vi "Get Stream State Register.vi"(6 "ready for output":bool=TRUE, 7 "stream state register":T2) -> (1 "output updated":bool caption="output valid", 2 "stream.state":T1)   [LabVIEW 2015, in "niInstr Streaming v1 FPGA.lvlib"]
uses:
  <instrlib>/_niInstr/Streaming/v1/FPGA/niInstr Streaming v1 FPGA.lvlib
  <instrlib>/_niInstr/Streaming/v1/FPGA/Public/Stream State Register.ctl
  <instrlib>/_niInstr/Streaming/v1/Common/Stream State.ctl
  <vilib>/rvi/Emulation/niFpgaSctlEmulationGetInTimedLoop.vi
  <vilib>/rvi/DataTransferAndStorage/Container/Common/niFpgaContainerExecOnDevCompGetState.vi
  <vilib>/rvi/Emulation/niFpgaEmulationIsFPGAContextNoSignature.vi
  <vilib>/rvi/DataTransferAndStorage/Container/Common/niFpgaContainerGetUniqueNameForEmu.vi
  <vilib>/rvi/eio/common/nirviEmuReportErrorAndStop.vi
  <vilib>/rvi/Emulation/niFpgaProcessEmulError.vi
  <vilib>/rvi/DataTransferAndStorage/Container/XNode/niFpgaContainer.xnode
  <vilib>/rvi/DataTransferAndStorage/Handshake/Emulation/niFpgaHandshakeEmulationRefIn.vi
  <instrlib>/_niInstr/Streaming/v1/Common/niInstr Streaming v1 Common.lvlib
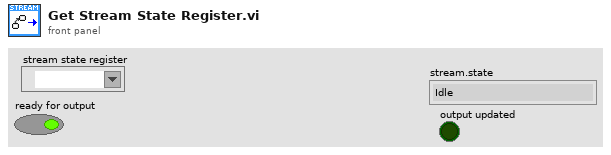
[diagram p1: front panel]
types:
  T1 = typedef "niInstr Streaming v1 Common.lvlib/Stream State.ctl" = enum8{"Idle", "Finite Transfer", "Continuous", "Done", "Error", "Not Ready", "Cancel"}
  T2 = typedef "niInstr Streaming v1 FPGA.lvlib/Stream State Register.ctl" = refnum<k21>
  T3 = enum8{"Idle", "Finite Transfer", "Continuous", "Done", "Error", "Not Ready", "Cancel"}
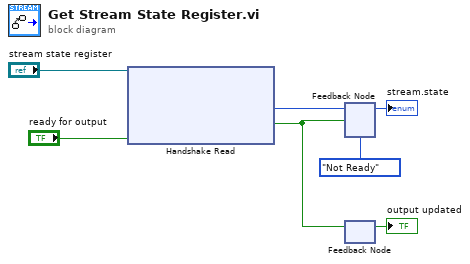
[diagram p0: block diagram]
diagram:
  n1 = xnode ("Handshake Read")("Ready for Output"="ready for output", "Handshake In"="stream state register") -> ("Data"=w4:T3, "Output Valid"=w2:bool)  [unwired: 1 out]
  n2 = feedback-in #1(w4, w2) -> ()
  n3 = feedback #1(Stream_State."Not Ready" ("stream.state")) -> (→"stream.state":T1)
  n4 = feedback #2() -> (→"output updated":bool)  [unwired: 1 in]
  n5 = feedback-in #2(w2) -> ()
